vi "FarfiledImageJoint3.vi"() -> ()   [LabVIEW 2018]
uses:
  <vilib>/vision/NI_Vision_Development_Module.lvlib
panel:
  out "俯仰":i32
  out "旋转":i32
  out "旋转":cluster{"俯仰":dbl, "旋转":dbl}
  out "俯仰":cluster{"俯仰":dbl, "旋转":dbl}
  out "俯仰":u8(slide) max=20 scale=0.0..172.0
  out "使用时间":u32[](array[numeric])
  out "返回":i32
  out "运行总时间s":dbl
  out "扫描进度":u8(slide) max=20 scale=0.0..172.0
  out "offset":i32[](array[numeric])
  out "Reference Grid":cluster{"数组":i32[], "数组":i32[]}
  out "时间":u32[](array[numeric])
  out "当前图像":T1(plugin-control)
  out "总图像":T1(plugin-control)
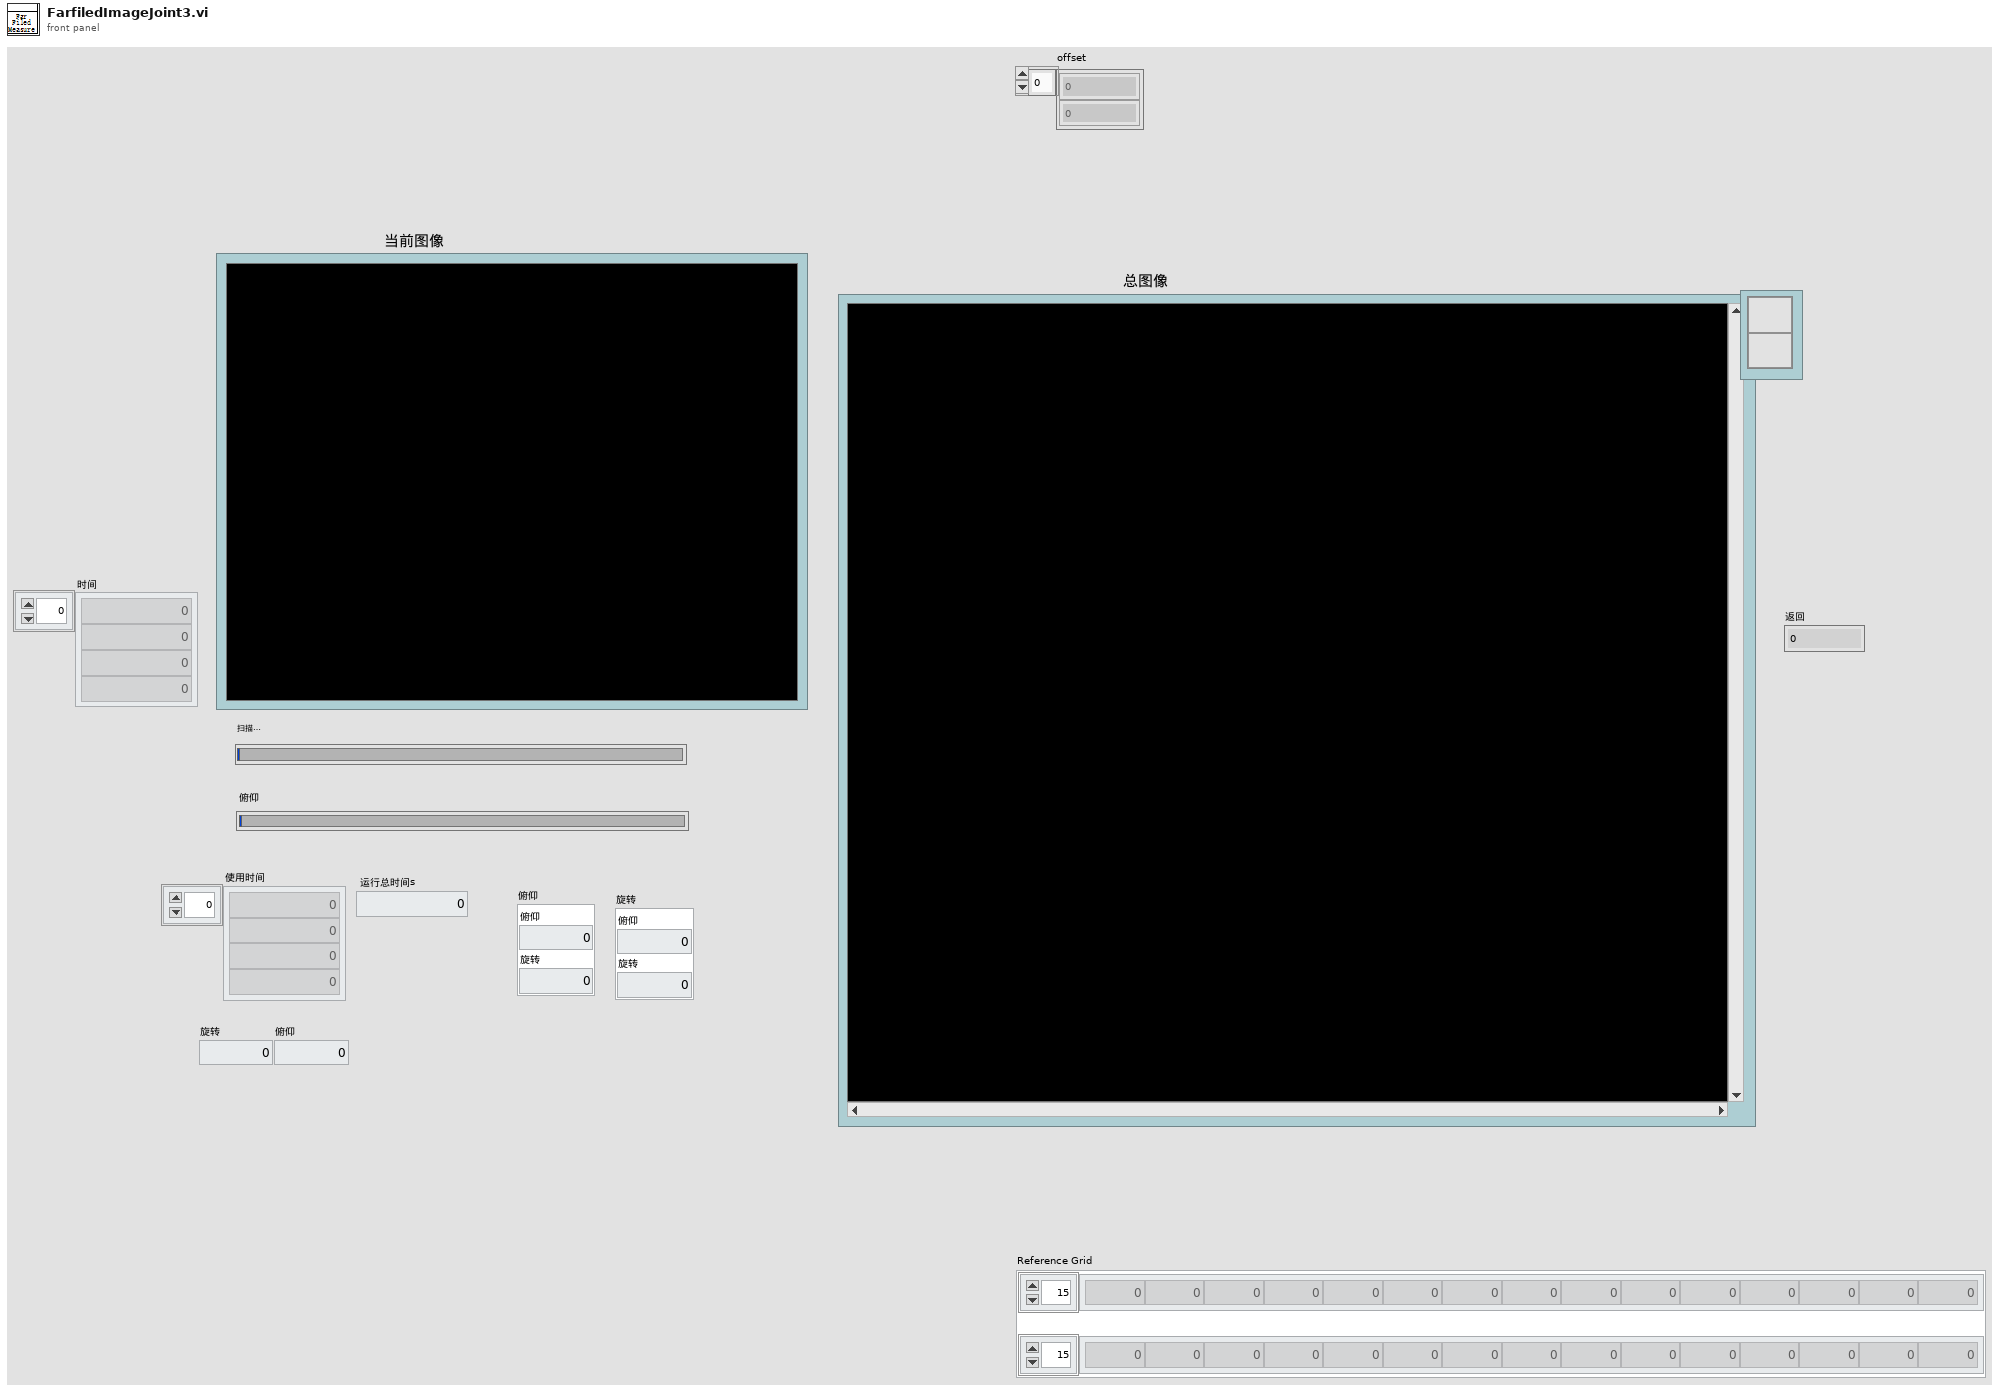
[diagram p1: front panel]
types:
  T1 = typedef "IMAQ Image.ctl" = refnum<image>
  T2 = typedef "控制电机枚举器.ctl" = enum16{"Z", "Y", "X", "发散角", "俯仰", "旋转"}
  T3 = typedef "Image Type" = u32
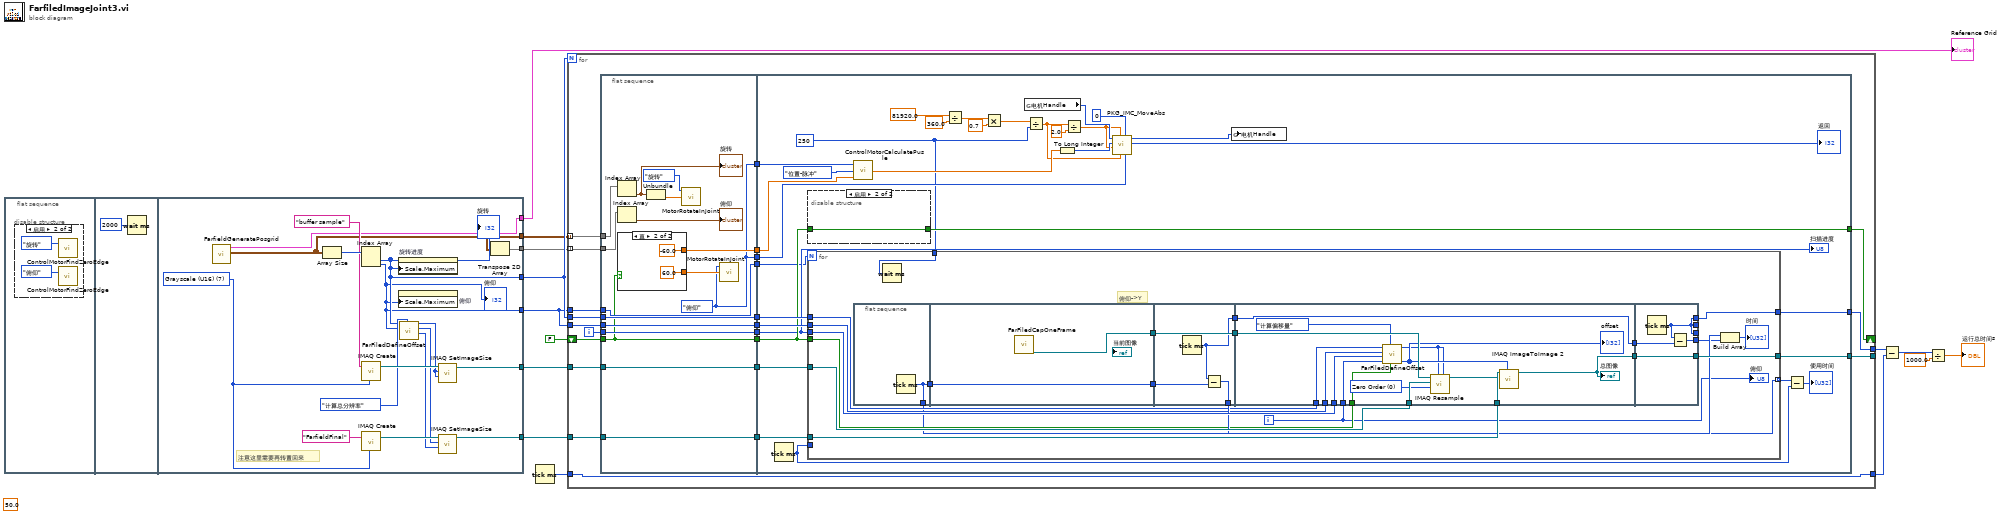
[diagram p0: block diagram]
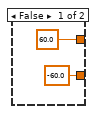
[diagram p3: hidden frame]
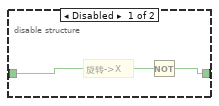
[diagram p4: hidden frame]
diagram:
  (unwired) 50.0
  n1 = flat-sequence {
    tunnel: [w28] -> w14
    tunnel: [w27] -> w13
    tunnel: [w26] -> w12
    tunnel: [w23] -> w4
    tunnel: [w18] -> w3
    tunnel: [w22] -> w2
    tunnel: [w21] -> w1
    frame #0 {
      n2 = disable-structure shown="启用" {
        frame Disabled {
        }
        frame Enabled {
          n3 = call "ControlMotorFindZeroEdge.vi"("控制电机"=控制电机枚举器."旋转") -> ()  [unwired: 2 in]
          n4 = call "ControlMotorFindZeroEdge.vi"("控制电机"=控制电机枚举器."俯仰") -> ()  [unwired: 2 in]
        }
      }
    }
    frame #1 {
      n5 = Wait (ms)(milliseconds to wait=u32 2000 ("等待时间（毫秒）")) -> ()  [unwired: 1 out]
    }
    frame #2 {
      w31 = T3 7 items=["Grayscale (U8)", "Grayscale (I16)", "Grayscale (SGL)", "Complex (CSG)", "RGB (U32)", "HSL (U32)", "RGB (U64)", "Grayscale (U16)"] ("Image Type")
      # "注意这里需要再转置回来"
      n6 = call "FarfieldGeneratePosgrid.vi"() -> ("posOut"=w22:cluster{"俯仰":dbl, "旋转":dbl}[][], "Reference Grid"=w26:cluster{"数组":i32[], "数组":i32[]})  [unwired: 9 in, 1 out]
      n7 = Array Size(array=w22) -> (size(s)=w34:i32[])
      n8 = Index Array(array=w34) -> (element #1=w23:i32, element #2=w18:i32)  [unwired: 2 in]
      "旋转" <- w23
      "俯仰" <- w18
      n9 = call "IMAQ Create"("Image Name"="buffer sample", "Image Type"=w31) -> ("New Image"=w29:T1)  [unwired: 3 in, 1 out]
      n10 = call "IMAQ Create"("Image Name"="FarfieldFinal", "Image Type"=w31) -> ("New Image"=w32:T1)  [unwired: 3 in, 1 out]
      n11 = property on="旋转进度" class="Slide (严格)"("Scale.Maximum"=w23) -> ()  [unwired: 2 in, 2 out]
      n12 = property on="俯仰" class="Slide (严格)"("Scale.Maximum"=w18) -> ()  [unwired: 2 in, 2 out]
      n13 = call "FarFiledDefineOffset.vi"("状态"=enum16{"计算总分辨率", "计算偏移量"}."计算总分辨率", "Y Pos Num"=w18, "X Pos Num"=w23) -> ("Y Resolution"=w19:i32, "X Resolution"=w20:i32, "单个分辨率"=w24:i32)  [unwired: 5 in, 1 out]
      n14 = call "IMAQ SetImageSize"("Y Resolution"=w24, "X Resolution"=w24, "Image"=w29) -> ("Image Out"=w28:T1)  [unwired: 2 in, 1 out]
      n15 = call "IMAQ SetImageSize"("Y Resolution"=w19, "X Resolution"=w20, "Image"=w32) -> ("Image Out"=w27:T1)  [unwired: 2 in, 1 out]
      n16 = Transpose 2D Array(2D array=w22) -> (transposed array=w21:cluster{"俯仰":dbl, "旋转":dbl}[][])
    }
  }
  n17 = Tick Count (ms)() -> (millisecond timer value=w10:u32)
  n18 = for {
    N: w4 -> [_]
    tunnel: w14 -> [w57]
    tunnel: w4 -> [w54]
    tunnel: w3 -> [w53]
    shift-right: [w52] -> _
    shift-left: FALSE -> [w51]
    tunnel: w13 -> [w55]
    tunnel: [w56] -> _
    tunnel: w10 -> [w48]
    tunnel: [w49] -> w9
    tunnel: [w48] -> w8
    tunnel: w3 -> [w47]
    tunnel: w2 -> [w36] mode=indexing
    tunnel: w1 -> [w35] mode=indexing
    i -> [w50]
    n19 = flat-sequence {
      tunnel: w47 -> [w68]
      tunnel: w50 -> [w69]
      tunnel: w51 -> [w67]
      tunnel: w53 -> [w70]
      tunnel: w54 -> [w71]
      tunnel: w55 -> [w72]
      tunnel: w57 -> [w73]
      tunnel: [w73] -> w46
      tunnel: [w72] -> w45
      tunnel: [w71] -> w44
      tunnel: [w70] -> w43
      tunnel: [w67] -> w42
      tunnel: [w69] -> w41
      tunnel: [w68] -> w40
      tunnel: [w64] -> w39
      tunnel: [w64] -> w38
      tunnel: [w65] -> w37
      tunnel: w36 -> [w62]
      tunnel: w35 -> [w59]
      tunnel: w46 -> [w109]
      tunnel: w45 -> [w107]
      tunnel: w44 -> [w106]
      tunnel: w43 -> [w105]
      tunnel: w42 -> [w103]
      tunnel: w41 -> [w102]
      tunnel: w40 -> [w100]
      tunnel: [w108] -> w56
      tunnel: [w104] -> w52
      tunnel: [w101] -> w49
      tunnel: w39 -> [w94]
      tunnel: w38 -> [w93]
      tunnel: w37 -> [w90]
      frame #0 {
        w64 = 控制电机枚举器."俯仰" ("控制电机")
        n20 = Index Array(array=w62) -> (element=w63:cluster{"俯仰":dbl, "旋转":dbl})  [unwired: 1 in]
        "旋转" <- w63
        n21 = Index Array(array=w59) -> (element=→"俯仰":cluster{"俯仰":dbl, "旋转":dbl})  [unwired: 1 in]
        n22 = case shown="真" w67 {
          tunnel: [-60.0 60.0 ("位置")] -> w66
          tunnel: [60.0 -60.0 ("数据")] -> w65
          frame False {
          }
          frame True {
          }
        }
        n23 = Unbundle(w63) -> ("旋转"=w60:dbl)  [unwired: 1 out]
        n24 = call "MotorRotateInJoint.vi"("位置"=w60, "axis"=控制电机枚举器."旋转" ("控制电机")) -> ()  [unwired: 2 in, 1 out]
        n25 = call "MotorRotateInJoint.vi"("位置"=w66, "axis"=w64) -> ()  [unwired: 2 in, 1 out]
      }
      frame #1 {
        w78 = u32 250 ("等待时间（毫秒）")
        n26 = Tick Count (ms)() -> (millisecond timer value=w88:u32)
        n27 = disable-structure shown="启用" {
          disable-tunnel: [w111 w112] -> w104
          disable-tunnel: w103 -> [w110 w112]
          frame Disabled {
            # "旋转->X"
            n28 = Not(x=w110) -> (.not. x?=w111:bool)
          }
          frame Enabled {
          }
        }
        n29 = for {
          N: w100 -> [_]
          tunnel: w109 -> [w133]
          tunnel: w102 -> [w130]
          tunnel: w106 -> [w126]
          tunnel: w105 -> [w125]
          tunnel: w103 -> [w124]
          tunnel: w107 -> [w131]
          tunnel: [w132] -> w108
          tunnel: [w116] -> w101
          tunnel: w88 -> [_]
          tunnel: [w115] -> w89 mode=indexing
          tunnel: w78 -> [w113]
          i -> [w114]
          # "俯仰->Y"
          n30 = flat-sequence {
            tunnel: [w134] -> w123
            tunnel: [w134] -> w115
            tunnel: [w136] -> w122
            tunnel: w123 -> [w135]
            tunnel: [w135] -> w121
            tunnel: w122 -> [w140]
            tunnel: [w140] -> w120
            tunnel: [w138] -> w119
            tunnel: w121 -> [w139]
            tunnel: [w137] -> w129
            tunnel: w133 -> [w155]
            tunnel: w131 -> [w153]
            tunnel: w120 -> [w150]
            tunnel: w119 -> [w149]
            tunnel: [w152] -> w118
            tunnel: [w149] -> w117
            tunnel: w126 -> [w148]
            tunnel: w125 -> [w147]
            tunnel: w130 -> [w141]
            tunnel: w114 -> [w142]
            tunnel: w124 -> [w145]
            tunnel: [w159] -> w132
            tunnel: w118 -> [w159]
            tunnel: w117 -> [w158]
            tunnel: [w157] -> w128
            tunnel: [w156] -> _
            tunnel: [w156] -> w116
            tunnel: [w156] -> _
            frame #0 {
              n31 = Tick Count (ms)() -> (millisecond timer value=w134:u32)
            }
            frame #1 {
              n32 = call "FarFiledCapOneFrame.vi"() -> ("Image_Normal"=w136:T1)  [unwired: 11 in]
            }
            frame #2 {
              n33 = Tick Count (ms)() -> (millisecond timer value=w138:u32)
              n34 = Subtract(x=w138, y=w139) -> (x-y=w137:u32)
            }
            frame #3 {
              w154 = u32 0 items=["Zero Order", "Bi-Linear", "Quadratic", "Cubic Spline"] ("Interpolation Type")
              n35 = call "FarFiledDefineOffset.vi"("正序？"=w145, "状态"=enum16{"计算总分辨率", "计算偏移量"}."计算偏移量", "当前Y位置"=w142, "当前X位置"=w141, "Y Pos Num"=w147, "X Pos Num"=w148) -> ("offset"=w144:i32[], "单个分辨率"=w143:i32)  [unwired: 2 in, 2 out]
              "offset" <- w144
              n36 = call "IMAQ Resample"("X Resolution"=w143, "Y Resolution"=w143, "Interpolation Type"=w154, "Image Dst"=w155, "Image Src"=w150) -> ("Image Dst Out"=w151:T1)  [unwired: 5 in, 1 out]
              n37 = call "IMAQ ImageToImage 2"("Offset Left/Top"=w144, "Image Src (Small)"=w151, "Image Src (Large)"=w153) -> ("Image Dst Out"=w152:T1)  [unwired: 7 in, 1 out]
              "总图像" <- w152
            }
            frame #4 {
              n38 = Tick Count (ms)() -> (millisecond timer value=w156:u32)
              n39 = Subtract(x=w156, y=w158) -> (x-y=w157:u32)
            }
          }
          n40 = Wait (ms)(milliseconds to wait=w113) -> ()  [unwired: 1 out]
          n41 = Build Array(w129, w128) -> (→"时间":u32[])
          "俯仰" <- w114
        }
        n42 = call "ControlMotorCalculatePusle.vi"("数据"=w90, "计算状态"=enum32{"位置-脉冲", "脉冲-位置"}."位置-脉冲", "控制电机"=w93) -> ("dataout"=w91:dbl)  [unwired: 2 in]
        n43 = Divide(x=81920.0, y=360.0) -> (x/y=w84:dbl)
        n44 = Multiply(x=w84, y=0.7) -> (x*y=w82:dbl)
        n45 = global read "参数.vi" "电机Handle"() -> (w98:u32)
        n46 = Divide(x=w82, y=w78) -> (x/y=w81:dbl)
        n47 = To Long Integer(number=w91) -> (32bit integer=w99:i32)
        n48 = Divide(x=w81, y=2.0) -> (x/y=w79:dbl)
        n49 = call "PKG_IMC_MoveAbs.vi"("axis"=w94, "wait"=0, "tgvel"=w81, "endvel"=w79, "startvel"=w79, "pos"=w99, "handle"=w98) -> ("function return"=→"返回":i32, "handle out"=w95:u32)  [unwired: 3 in]
        n50 = global write "参数.vi" "电机Handle"(w95) -> ()
        n51 = Subtract(x=w89, y=w88) -> (x-y=→"使用时间":u32[])
        "扫描进度" <- w102
      }
    }
  }
  n52 = Subtract(x=w9, y=w8) -> (x-y=w7:u32)
  n53 = Divide(x=w7, y=1000.0) -> (x/y=→"运行总时间s":dbl)
  "Reference Grid" <- w12
